vi "counter_channel_producer.vi"(7 "Channel":i32, 8 "error in (no error)":errorcluster, 9 "aData Out":dbl[][](array[numeric]), 10 "Queue in":refnum<queue>, 11 "output cluster in":T1) -> (0 "error out":errorcluster, 3 "output cluster out":T1)   [LabVIEW 2025, in "LabJackEKG.lvlib"]
uses:
  LabJackEKG.lvlib
  Tests/StreamProducerLoopData.ctl
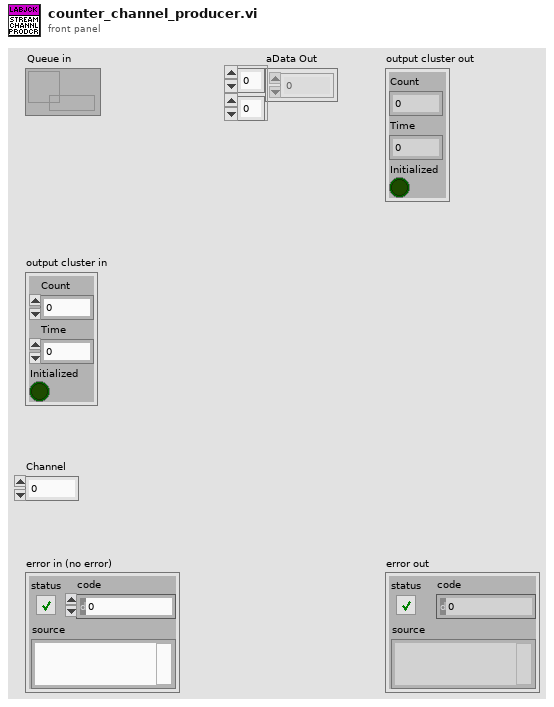
[diagram p1: front panel]
types:
  T1 = typedef "LabJackEKG.lvlib/StreamProducerLoopData.ctl" = cluster{"Count":i64, "Time":i64, "Initialized":bool}
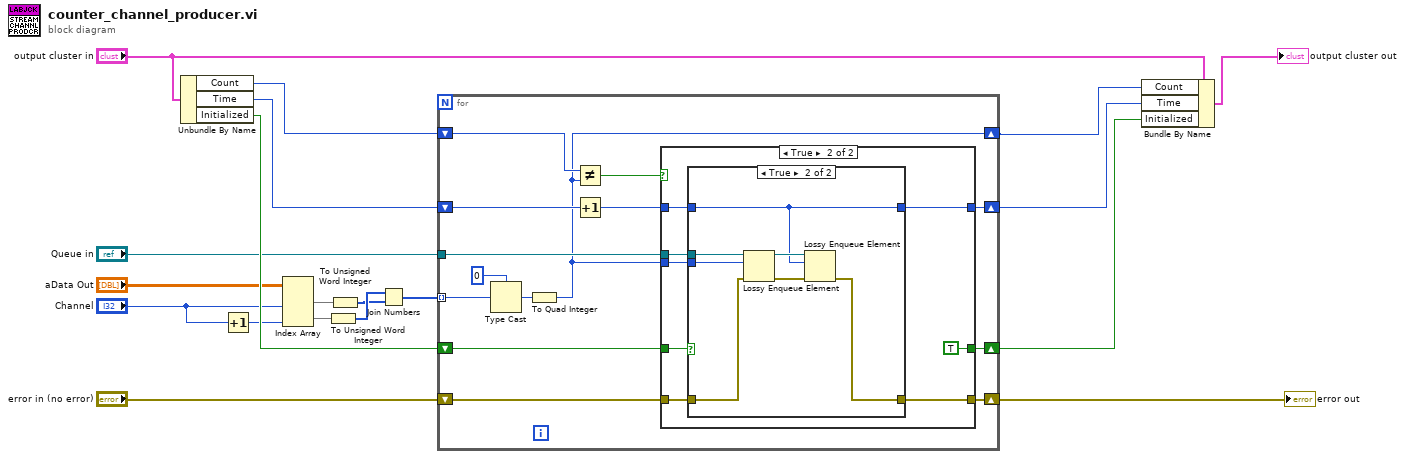
[diagram p0: block diagram]
diagram:
  n1 = Unbundle By Name("output cluster in") -> ("Count"=w19:i64, "Time"=w18:i64, "Initialized"=w17:bool)
  n2 = Increment(x="Channel") -> (x+1=w4:i32)
  n3 = Index Array(array="aData Out", index (col) #1="Channel", index (col) #2=w4) -> (element #1=w7:dbl[], element #2=w11:dbl[])  [unwired: 2 in]
  n4 = To Unsigned Word Integer(number=w11) -> (unsigned 16bit integer=w3:u16[])
  n5 = To Unsigned Word Integer(number=w7) -> (unsigned 16bit integer=w2:u16[])
  n6 = Join Numbers(hi=w3, lo=w2) -> ((hi.lo)=w1:u32[])
  n7 = for {
    tunnel: w1 -> [w27] mode=indexing
    tunnel: "Queue in" -> [w33]
    shift-right: [w32] -> w10
    shift-left: "error in (no error)" -> [w31]
    shift-right: [w30] -> w13
    shift-left: w18 -> [w29]
    shift-right: [w20] -> w12
    shift-left: w19 -> [w28]
    shift-right: [w25] -> w14
    shift-left: w17 -> [w24]
    n8 = Type Cast(type=0, x=w27) -> (*(type *) &x=w22:i32)
    n9 = To Quad Integer(1:w22) -> (0:w20:i64)
    n10 = Not Equal?(x=w28, y=w20) -> (x != y?=w23:bool)
    n11 = Increment(x=w29) -> (x+1=w26:i64)
    n12 = case shown="True" w23 {
      tunnel: w33 -> [_ w44]
      tunnel: [w36 w41] -> w32
      tunnel: w31 -> [w36 w43]
      tunnel: w20 -> [_ w42]
      tunnel: [w35 w37] -> w30
      tunnel: w26 -> [w35 w40]
      tunnel: [w34 TRUE] -> w25
      tunnel: w24 -> [w34 w38]
      frame False {
      }
      frame True {
        n13 = case shown="True" w38 {
          tunnel: w44 -> [_ w53]
          tunnel: w43 -> [w46 w51]
          tunnel: w42 -> [_ w50]
          tunnel: [w46 w49] -> w41
          tunnel: w40 -> [w45 w47]
          tunnel: [w45 w47] -> w37
          frame False {
          }
          frame True {
            n14 = Lossy Enqueue Element(queue=w53, element=w50, error in (no error)=w51) -> (queue out=w48:refnum<queue>, error out=w52:errorcluster)  [unwired: 2 out]
            n15 = Lossy Enqueue Element(queue=w48, element=w47, error in (no error)=w52) -> (error out=w49:errorcluster)  [unwired: 3 out]
          }
        }
      }
    }
  }
  "error out" <- w10
  n16 = Bundle By Name(cluster="output cluster in", "Count"=w12, "Time"=w13, "Initialized"=w14) -> (→"output cluster out":T1)
